vi "Initialize.vi"(8 "error in (no error)":errorcluster, 11 "Test 1 in":refnum<class "Test 1.lvclass">) -> (0 "error out":errorcluster, 3 "Test 1 out":refnum<class "Test 1.lvclass">)   [LabVIEW 2020, in "Scratchpad.lvlib" / "Test 1.lvlib" / "Test 1.lvclass"]
uses:
  Test 1.lvclass
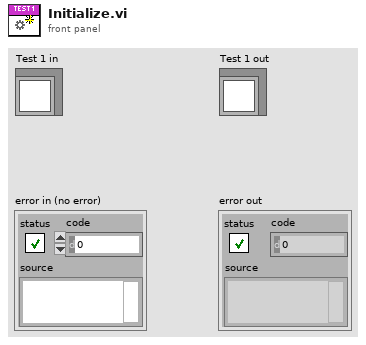
[diagram p1: front panel]
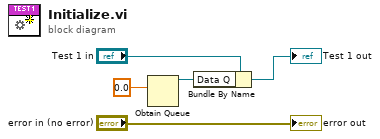
[diagram p0: block diagram]
diagram:
  n1 = Obtain Queue(element data type=0.0) -> (queue out=w1:refnum<queue>)  [unwired: 4 in, 2 out]
  n2 = Bundle By Name(cluster="Test 1 in", "Data Q"=w1) -> (→"Test 1 out":refnum<class "Test 1.lvclass">)
  "error out" <- "error in (no error)"
